vi "RFFE Compile Pattern.vi"(0 "Destination Directory":path, 1 "Alias":string, 5 "Slave Address":T4=12 format="%02x", 7 "Register Address":T1 format="%02x", 9 "Register Data":T3[](array[typedef]) format="%02x", 11 "error in (no error)":errorcluster, 12 "Byte Count":i32=1, 13 "Command Type":T2) -> (4 "Compiled Pattern Path":path, 15 "error out":errorcluster)   [LabVIEW 2018]
uses:
  Slave Address.ctl
  Register Data.ctl
  Command Type.ctl
  Register Address.ctl
  Exports/Generate Register 0 Write Vectors.vi
  Exports/Generate Register Write Vectors.vi
  Exports/Generate Extended Register Read Long Vectors.vi
  Exports/Generate Register Read Vectors.vi
  Exports/Generate Extended Register Read Vectors.vi
  Exports/Generate Extended Register Write Vectors.vi
  Exports/Generate Extended Register Write Long Vectors.vi
  MIPI RFFE API.lvlib
panel:
  in  "Delete Source File":bool=TRUE
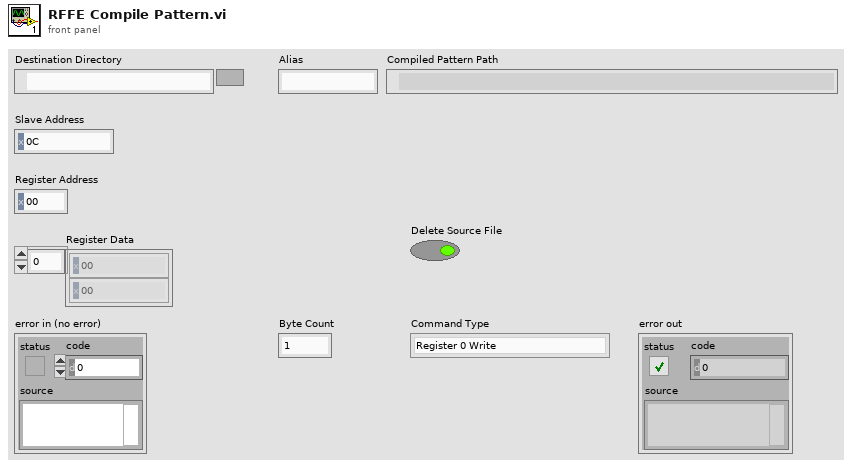
[diagram p1: front panel]
types:
  T1 = typedef "MIPI RFFE API.lvlib/Register Address.ctl" = u16
  T2 = typedef "MIPI RFFE API.lvlib/Command Type.ctl" = enum16{"Register 0 Write", "Register Write", "Extended Register Write", "Extended Register Write Long", "Register Read", "Extended Register Read", "Extended Register Read Long"}
  T3 = typedef "MIPI RFFE API.lvlib/Register Data.ctl" = u8
  T4 = typedef "MIPI RFFE API.lvlib/Slave Address.ctl" = u8
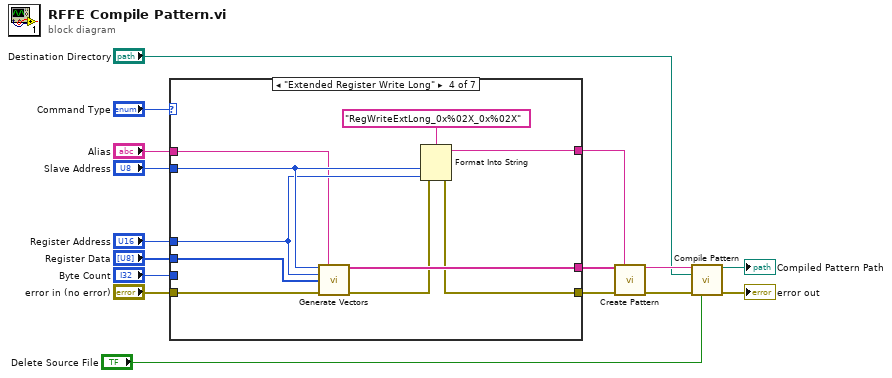
[diagram p0: block diagram]
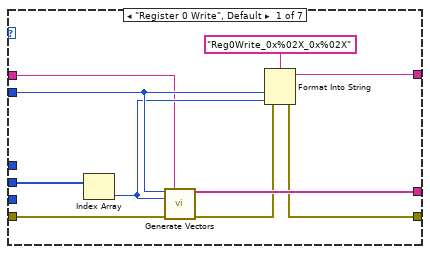
[diagram p2: hidden frame]
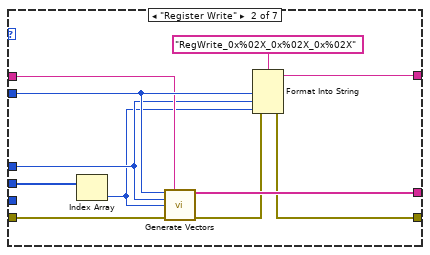
[diagram p3: hidden frame]
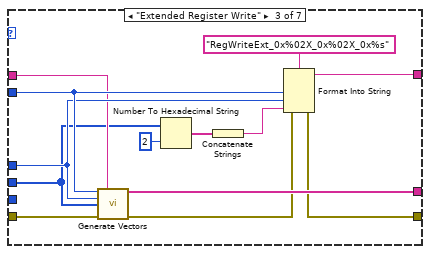
[diagram p4: hidden frame]
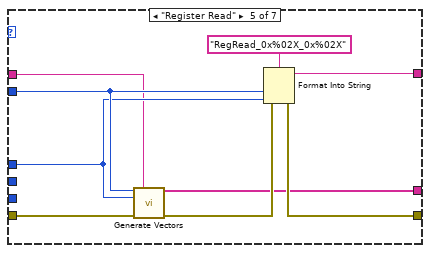
[diagram p5: hidden frame]
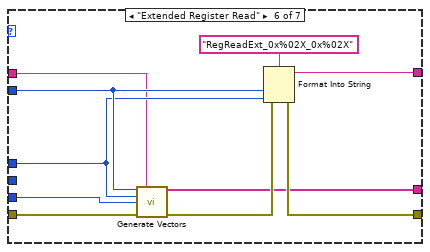
[diagram p6: hidden frame]
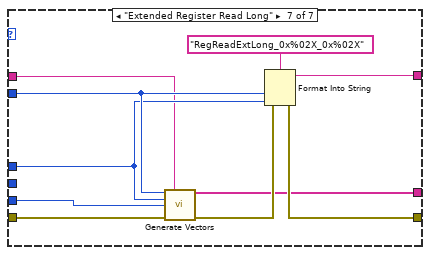
[diagram p7: hidden frame]
diagram:
  n1 = case shown="\"Extended Register Write Long\"" "Command Type" {
    tunnel: [w26 w37 w50 w60 w63 w73 w83] -> w5
    tunnel: [w24 w35 w48 w58 w68 w78 w88] -> w14
    tunnel: [w23 w34 w47 w57 w67 w77 w87] -> w3
    tunnel: "Slave Address" -> [w21 w32 w45 w55 w65 w75 w85]
    tunnel: "Register Data" -> [w20 w31 w41 w53 _ _ _]
    tunnel: "Register Address" -> [_ w28 w44 w54 w64 w74 w84]
    tunnel: "error in (no error)" -> [w18 w30 w43 w52 w62 w72 w82]
    tunnel: "Alias" -> [w17 w29 w42 w51 w61 w71 w81]
    tunnel: "Byte Count" -> [_ _ _ _ _ w70 w80]
    frame "Register 0 Write", Default {
      n2 = Index Array(array=w20) -> (element=w19:T3)  [unwired: 1 in]
      n3 = call-poly "Generate Vectors.vi"("Slave Address"=w21, "Alias"=w17, "Register Data"=w19, "error in (no error)"=w18) -> ("Vector Statements"=w26:string[], "error out"=w25:errorcluster)  [unwired: 10 in]
      n4 = Format Into String(format string="Reg0Write_0x%02X_0x%02X" ("Name"), error in=w25, w21, w19) -> (resulting string=w23:string, error out=w24:errorcluster)  [unwired: 1 in]
    }
    frame "Register Write" {
      n5 = Index Array(array=w31) -> (element=w27:T3)  [unwired: 1 in]
      n6 = call-poly "Generate Vectors.vi"("Slave Address"=w32, "Alias"=w29, "Register Address"=w28, "Register Data"=w27, "error in (no error)"=w30) -> ("Vector Statements"=w37:string[], "error out"=w36:errorcluster)  [unwired: 9 in]
      n7 = Format Into String(format string="RegWrite_0x%02X_0x%02X_0x%02X" ("Name"), error in=w36, w32, w28, w27) -> (resulting string=w34:string, error out=w35:errorcluster)  [unwired: 1 in]
    }
    frame "Extended Register Write" {
      n8 = call-poly "Generate Vectors.vi"("Slave Address"=w45, "Alias"=w42, "Register Address"=w44, "Register Data"=w41, "error in (no error)"=w43) -> ("Vector Statements"=w50:string[], "error out"=w49:errorcluster)  [unwired: 9 in]
      n9 = Number To Hexadecimal String(1:i16 2 ("width (-)"), 2:w41) -> (0:w40:string[])
      n10 = Concatenate Strings(w40) -> (w39:string)
      n11 = Format Into String(format string="RegWriteExt_0x%02X_0x%02X_0x%s" ("Name"), error in=w49, w45, w44, w39) -> (resulting string=w47:string, error out=w48:errorcluster)  [unwired: 1 in]
    }
    frame "Extended Register Write Long" {
      n12 = call-poly "Generate Vectors.vi"("Slave Address"=w55, "Alias"=w51, "Register Address"=w54, "Register Data"=w53, "error in (no error)"=w52) -> ("Vector Statements"=w60:string[], "error out"=w59:errorcluster)  [unwired: 9 in]
      n13 = Format Into String(format string="RegWriteExtLong_0x%02X_0x%02X" ("Name"), error in=w59, w55, w54) -> (resulting string=w57:string, error out=w58:errorcluster)  [unwired: 1 in]
    }
    frame "Register Read" {
      n14 = call-poly "Generate Vectors.vi"("Slave Address"=w65, "Alias"=w61, "Register Address"=w64, "error in (no error)"=w62) -> ("Vector Statements"=w63:string[], "error out"=w69:errorcluster)  [unwired: 10 in]
      n15 = Format Into String(format string="RegRead_0x%02X_0x%02X" ("Name"), error in=w69, w65, w64) -> (resulting string=w67:string, error out=w68:errorcluster)  [unwired: 1 in]
    }
    frame "Extended Register Read" {
      n16 = call-poly "Generate Vectors.vi"("Slave Address"=w75, "Alias"=w71, "Register Address"=w74, "Byte Count"=w70, "error in (no error)"=w72) -> ("Vector Statements"=w73:string[], "error out"=w79:errorcluster)  [unwired: 9 in]
      n17 = Format Into String(format string="RegReadExt_0x%02X_0x%02X" ("Name"), error in=w79, w75, w74) -> (resulting string=w77:string, error out=w78:errorcluster)  [unwired: 1 in]
    }
    frame "Extended Register Read Long" {
      n18 = call-poly "Generate Vectors.vi"("Slave Address"=w85, "Alias"=w81, "Register Address"=w84, "Byte Count"=w80, "error in (no error)"=w82) -> ("Vector Statements"=w83:string[], "error out"=w89:errorcluster)  [unwired: 9 in]
      n19 = Format Into String(format string="RegReadExtLong_0x%02X_0x%02X" ("Name"), error in=w89, w85, w84) -> (resulting string=w87:string, error out=w88:errorcluster)  [unwired: 1 in]
    }
  }
  n20 = call "Create Pattern.vi"("Vector Statements"=w5, "Name"=w3, "error in (no error)"=w14) -> ("Digital Pattern"=w4:string, "error out"=w6:errorcluster)  [unwired: 11 in]
  n21 = call "Compile Pattern.vi"("Digital Pattern"=w4, "Destination"="Destination Directory", "error in (no error)"=w6, "Delete Source File"="Delete Source File") -> ("Compiled Pattern Path"=→"Compiled Pattern Path":path, "error out"=→"error out":errorcluster)  [unwired: 10 in]
